vi "Pos_modifi.vi"() -> ()   [LabVIEW 2020]
panel:
  in  "Pos_modif":T1
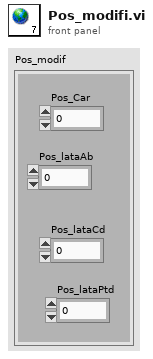
[diagram p1: front panel]
types:
  T1 = cluster{"Pos_Car":dbl, "Pos_lataAb":dbl, "Pos_lataCd":dbl, "Pos_lataPtd":dbl}
diagram:
